vi "VolumeKnobGlobal.vi"() -> ()   [LabVIEW 2016]
panel:
  out "Volume":dbl
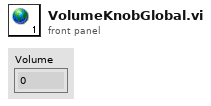
[diagram p1: front panel]
diagram:
